vi "Compare Ch with Ch List.vi"(8 "error in (no error)":errorcluster, 10 "Compare List":refnum<class "ChannelVS.lvclass">[](array[class]), 11 "Channel to compare":refnum<class "ChannelVS.lvclass">) -> (0 "error out":errorcluster, 3 "Channel out":refnum<class "ChannelVS.lvclass">)   [LabVIEW 2021, in "Shared Variables CD 2.0 Configuration.lvlib" / "ChannelVS.lvclass"]
uses:
  ChannelVS.lvclass
  ChannelVS.lvclass/ChannelVS.ctl
  OneDrive - NI/Documents/GitHub/Shared-Variable-Custom-Device-2.0/Modules/Channel.lvlibp/Channel.lvclass
  OneDrive - NI/Documents/GitHub/Shared-Variable-Custom-Device-2.0/Modules/Channel.lvlibp/1abvi3w/vi.lib/Utility/Data Type/Type Definitions/Data Type.ctl
  OneDrive - NI/Documents/GitHub/Shared-Variable-Custom-Device-2.0/Modules/Channel.lvlibp/1abvi3w/vi.lib/Utility/Data Type/NI_Data Type.lvlib
  <vilib>/NI VeriStand/Custom Device API/Custom Device Item Ref.ctl
  <vilib>/NI VeriStand/Custom Device API/Custom Device API.lvlib
  C:/Users/NPowley/OneDrive - NI/Documents/GitHub/Shared-Variable-Custom-Device-2.0/Modules/Channel.lvlibp/Channel.lvclass
  C:/Users/NPowley/Downloads/Shared-Variable-Custom-Device-2.0-master (8)/Shared-Variable-Custom-Device-2.0-master/Source_2017/Source/Shared Variables CD 2.0/Configuration/Support/ChannelVS/ChannelVS.lvclass
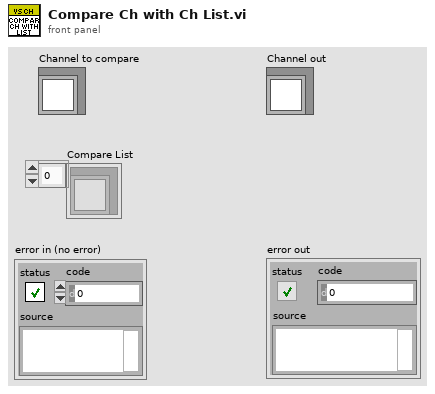
[diagram p1: front panel]
types:
  T1 = typedef "Custom Device API.lvlib/Custom Device Item Ref.ctl" = u64
  T2 = typedef "Channel.lvlibp/NI_Data Type.lvlib/Data Type.ctl" = enum8{"Invalid Type", "Void", "I8", "I16", "I32", "I64", "U8", "U16", "U32", "U64", "Single Float", "Double Float", "Extended Float", "Single Complex", "Double Complex", "Extended Complex", "Enum U8", "Enum U16", "Enum U32", "Enum U64", "Single Float With Unit", "Double Float With Unit", "Extended Float With Unit", "Single Complex with Unit", "Double Complex with Unit", "Extended Complex with Unit", "Boolean", "String", "Path", "Picture", "Tag", "Array", "Cluster", "Variant", "LV Variant", "Waveform", "Timestamp", "Digital Waveform", "Digital Data", "ExpressData", "Refnum", "External Data", "VI", "Poly VI", "LabVIEW Class Instance", "Fixed Point", "Set Collection", "Map Collection"}
  T3 = cluster{"Name":string, "URL":string, "DataType":T2}
  T4 = cluster{"Name":bool, "URL":bool, "DataType":bool}
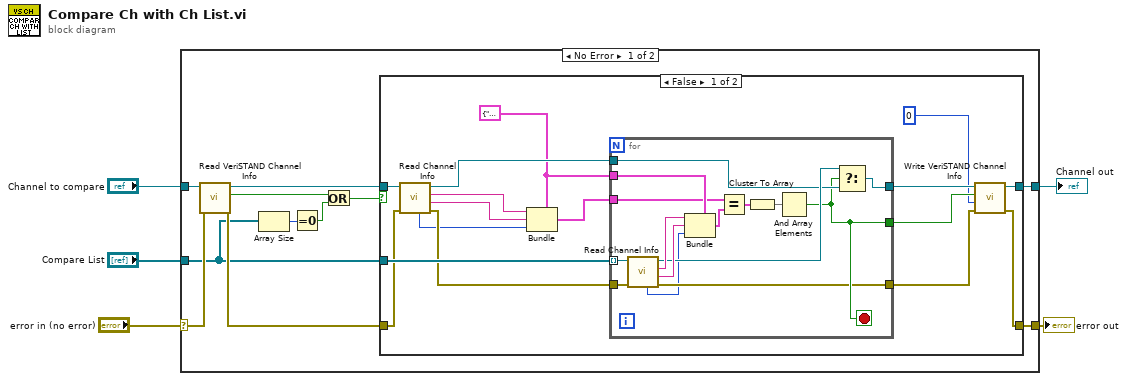
[diagram p0: block diagram]
diagram:
  n1 = case shown="No Error" "error in (no error)" {
    selector: "error in (no error)" -> [w12 w51]
    tunnel: "Compare List" -> [w9 _]
    tunnel: [w16 w50] -> w4
    tunnel: "Channel to compare" -> [w15 w50]
    tunnel: [w10 w51] -> w1
    frame No Error {
      n2 = call "Read VeriSTAND Channel Info.vi"("error in (no error)"=w12, "ChannelVS in"=w15) -> ("error out"=w11:errorcluster, "Exist in VeriSTAND"=w13:bool, "ChannelVS out"=w14:refnum<class "ChannelVS.lvclass">)  [unwired: 6 in, 1 out]
      n3 = Array Size(array=w9) -> (size(s)=w7:i32)
      n4 = Equal To 0?(x=w7) -> (x = 0?=w6:bool)
      n5 = Or(x=w13, y=w6) -> (x .or. y?=w8:bool)
      n6 = case shown="False" w8 {
        tunnel: w9 -> [w32 _]
        tunnel: [w28 w49] -> w16
        tunnel: w14 -> [w25 w49]
        tunnel: w11 -> [w24 w48]
        tunnel: [w21 w48] -> w10
        frame False {
          w29 = T3 {"Name"="", "URL"="", "DataType"=enum."Invalid Type"} ("cluster")
          n7 = call "Read Channel Info.vi"("error in (no error)"=w24, "Channel in"=w25) -> ("error out"=w23:errorcluster, "URL"=w18:string, "Name"=w19:string, "Channel out"=w30:refnum<class "ChannelVS.lvclass">, "DataType"=w17:T2)  [unwired: 4 in, 1 out]
          n8 = Bundle(cluster=w29, "Name"=w19, "URL"=w18, "DataType"=w17) -> (w31:T3)
          n9 = for {
            tunnel: w32 -> [w47] mode=indexing
            tunnel: w31 -> [w42]
            tunnel: w29 -> [w44]
            tunnel: w30 -> [w38]
            tunnel: [w37] -> w26
            tunnel: [w36] -> w27
            tunnel: w23 -> [w35]
            tunnel: [w34] -> w22
            stop <- w36 stop-if-true
            n10 = call "Read Channel Info.vi"("error in (no error)"=w35, "Channel in"=w47) -> ("error out"=w34:errorcluster, "URL"=w45:string, "Name"=w46:string, "Channel out"=w39:refnum<class "ChannelVS.lvclass">, "DataType"=w33:T2)  [unwired: 4 in, 1 out]
            n11 = Bundle(cluster=w44, "Name"=w46, "URL"=w45, "DataType"=w33) -> (w43:T3)
            n12 = Equal?(x=w42, y=w43) -> (x = y?=w41:T4)
            n13 = Cluster To Array(cluster=w41) -> (array=w40:bool[])
            n14 = And Array Elements(Boolean array=w40) -> (logical AND=w36:bool)
            n15 = Select(t=w39, s=w36, f=w38) -> (s? t:f=w37:refnum<class "ChannelVS.lvclass">)
          }
          n16 = call "Write VeriSTAND Channel Info.vi"("error in (no error)"=w22, "VeriSTAND Reference"=T1 0, "Exist in VeriSTAND"=w27, "ChannelVS in"=w26) -> ("error out"=w21:errorcluster, "ChannelVS out"=w28:refnum<class "ChannelVS.lvclass">)  [unwired: 6 in]
        }
        frame True {
        }
      }
    }
    frame Error {
    }
  }
  "Channel out" <- w4
  "error out" <- w1
